vi "poly_is_either_run_ref.vi"(4 "vi ref":refnum<vi>) -> (1 "is running?":bool)   [LabVIEW 2015]
uses:
  poly_is_running_state.vi
  poly_is_running_top_level_state.vi
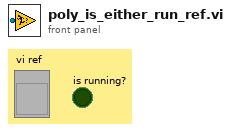
[diagram p1: front panel]
types:
  T1 = enum32{"Bad", "Idle", "Run top level", "Running"}
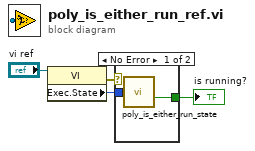
[diagram p0: block diagram]
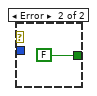
[diagram p2: hidden frame]
diagram:
  n1 = property class="VI"(reference="vi ref") -> (error out=w1:errorcluster, "Exec.State"=w3:T1)  [unwired: 1 in, 1 out]
  n2 = case shown="No Error" w1 {
    tunnel: w3 -> [w6 _]
    tunnel: [w5 FALSE] -> w2
    frame No Error {
      n3 = call "poly_is_either_run_state.vi"("execution state"=w6) -> ("is running?"=w5:bool)  [unwired: 4 in]
    }
    frame Error {
    }
  }
  "is running?" <- w2
